vi "CAN Test Max number of frames.vi"() -> ()   [LabVIEW 2025]
uses:
  <vilib>/xnet/xnet.llb/XNET Frame CAN.ctl
  <vilib>/xnet/xnet.llb/XNET Frame Type CAN.ctl
  <vilib>/xnet/xnet.llb/XNET Create Session (Frame Output Stream).vi
  <vilib>/xnet/xnet.llb/XNET Write (Frame CAN).vi
  <resource>/objmgr/xnet.rc
panel:
  in  "Number ot Frames":i32=10000
  out "Frame Number":i32
  in  "Echo Transmit":bool
  in  "Wait time (ms)":u32=1000
  in  "Baud Rate (bps)":u64=125000
  in  "Termination":bool
  in  "CAN interface":refnum<k21>
  # "Sends CAN messages to the selected interface with the selected rate (defualt is 1000 ms).\nSet \"Echo Trasmit\" to true when testing on the same interface what the plugin use."
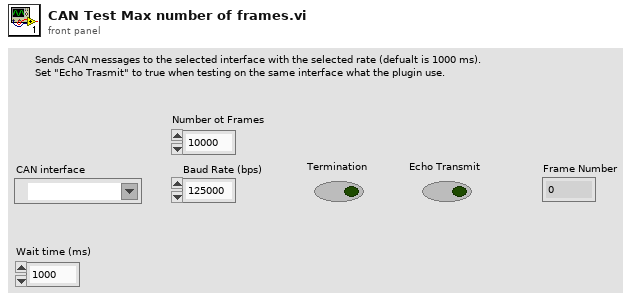
[diagram p1: front panel]
types:
  T1 = typedef "XNET Frame CAN.ctl" = cluster{"timestamp":timestamp, "payload":u8[], "identifier":u32, "type":T2, "extended?":bool, "echo?":bool}
  T2 = typedef "XNET Frame Type CAN.ctl" = u8
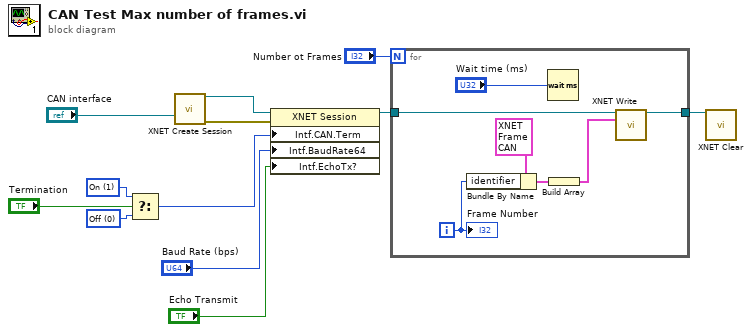
[diagram p0: block diagram]
diagram:
  w11 = u32 1 items=["Off", "On"] ("Interface:CAN:Termination")
  w12 = u32 0 items=["Off", "On"] ("Interface:CAN:Termination")
  n1 = Select(t=w11, s="Termination", f=w12) -> (s? t:f=w10:u32)
  n2 = call-poly <vilib>:"XNET Create Session.vi"("interface"="CAN interface") -> ("session out"=w8:refnum<k21>, "error out"=w9:errorcluster)  [unwired: 13 in]
  n3 = property class="XNET Session"(reference=w8, error in=w9, "Intf.CAN.Term"=w10, "Intf.BaudRate64"="Baud Rate (bps)", "Intf.EchoTx?"="Echo Transmit") -> (reference out=w4:refnum<k21>)  [unwired: 1 out]
  n4 = for {
    N: "Number ot Frames" -> [_]
    tunnel: w4 -> [w19]
    tunnel: [w18] -> w1
    i -> [w15]
    n5 = Bundle By Name(cluster=T1 {"timestamp"=timestamp(0 s since 1904-01-01), "payload"=[1, 2, 3, 4], "identifier"=257, "type"=0, "extended?"=FALSE, "echo?"=FALSE} ("CAN frame"), "identifier"=w15) -> (w13:T1)
    n6 = Wait (ms)(milliseconds to wait="Wait time (ms)") -> ()  [unwired: 1 out]
    n7 = Build Array(w13) -> (w14:T1[])
    n8 = call-poly <vilib>:"XNET Write.vi"("session in"=w19, "data"=w14) -> ("session out"=w18:refnum<k21>)  [unwired: 12 in, 1 out]
    "Frame Number" <- w15
  }
  n9 = call <vilib>:"XNET Clear.vi"("session in"=w1) -> ()  [unwired: 14 in, 1 out]
